vi "OnValueChange_AnyKey.vi"(8 "error in (no error)":errorcluster, 11 "SnakeDemo in":refnum<class "SnakeDemo.lvclass">) -> (0 "error out":errorcluster, 3 "SnakeDemo out":refnum<class "SnakeDemo.lvclass">)   [LabVIEW 2019, in "RT_Game.lvlib" / "SnakeDemo.lvclass"]
uses:
  SnakeDemo.lvclass
  SnakeGame/SnakeGame.lvclass
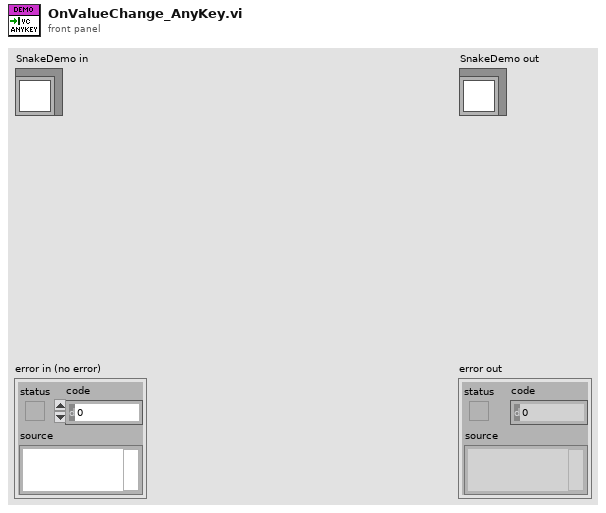
[diagram p1: front panel]
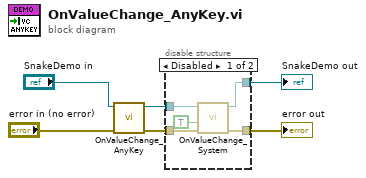
[diagram p0: block diagram]
diagram:
  n1 = call-parent "OnValueChange_AnyKey.vi"("error in (no error)"="error in (no error)", "Game in"="SnakeDemo in") -> ("error out"=w6:errorcluster, "Game out"=w2:refnum<class "SnakeDemo.lvclass">)  [unwired: 8 in]
  n2 = disable-structure shown="Disabled" {
    disable-tunnel: w6 -> [w11 w12]
    disable-tunnel: [w10 w12] -> w3
    disable-tunnel: w2 -> [w9 w13]
    disable-tunnel: [w8 w13] -> w1
    frame Disabled {
      n3 = call-dynamic "OnValueChange_System.vi"("error in (no error)"=w11, "Value"=TRUE, "SnakeGame in"=w9) -> ("error out"=w10:errorcluster, "SnakeGame out"=w8:refnum<class "SnakeDemo.lvclass">)  [unwired: 7 in]
    }
    frame Enabled {
    }
  }
  "error out" <- w3
  "SnakeDemo out" <- w1
